vi "Total Images.vi"(8 "Error in":errorcluster, 10 "Total Images":u32, 11 "Controller in":refnum<class "Controller.lvclass">) -> (0 "Error out":errorcluster, 3 "Controller out":refnum<class "Controller.lvclass">)   [LabVIEW 2022 SP3, in "Controller.lvlib" / "Controller.lvclass"]
uses:
  Controller.lvclass
  Controller.lvclass/Controller.ctl
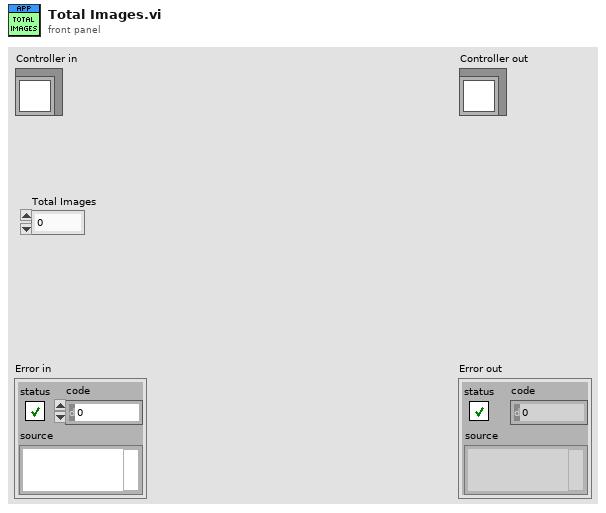
[diagram p1: front panel]
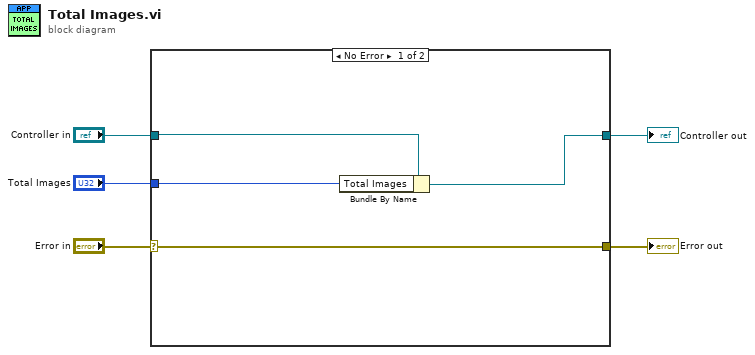
[diagram p0: block diagram]
diagram:
  n1 = case shown="No Error" "Error in" {
    selector: "Error in" -> [w9 w10]
    tunnel: "Controller in" -> [w8 w11]
    tunnel: [w7 w11] -> w4
    tunnel: [w9 w10] -> w3
    tunnel: "Total Images" -> [w6 _]
    frame No Error {
      n2 = Bundle By Name(cluster=w8, "Total Images"=w6) -> (w7:refnum<class "Controller.lvclass">)
    }
    frame Error {
    }
  }
  "Error out" <- w3
  "Controller out" <- w4
